vi "Initialize Waterfall Display for Octave.vi"(2 "colors":T2={"frame"=16763904, "plot"=52224, "background"=0}, 3 "display  bounds":T1={"left"=20, "top"=20, "width"=600, "heigth"=400} {"heigth" min=300; "width" min=400}, 4 "window title":string="Octave waterfall") -> (0 "error out":errorcluster, 1 "waterfall ref":refnum<vi>)   [LabVIEW 2017]
doc: "Initializes the waterfall display to display octave spectra and generates a waterfall reference to use to send data to this display or to close the display. This VI also specifies the title, colors and display bounds of the waterfall display. This VI does not open the waterfall display. The waterfall display opens when it receives its first data from Send Data to Waterfall for Octave VI."
uses:
  <vilib>/addons/Sound and Vibration/compatibility/Waterfall/subVIs/sv_Waterfall for Octave Global.vi
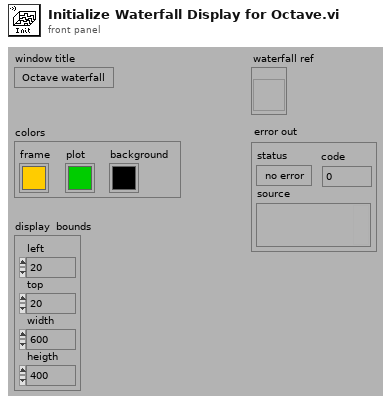
[diagram p1: front panel]
types:
  T1 = cluster{"left":i16, "top":i16, "width":i16, "heigth":i16}
  T2 = cluster{"frame":u32, "plot":u32, "background":u32}
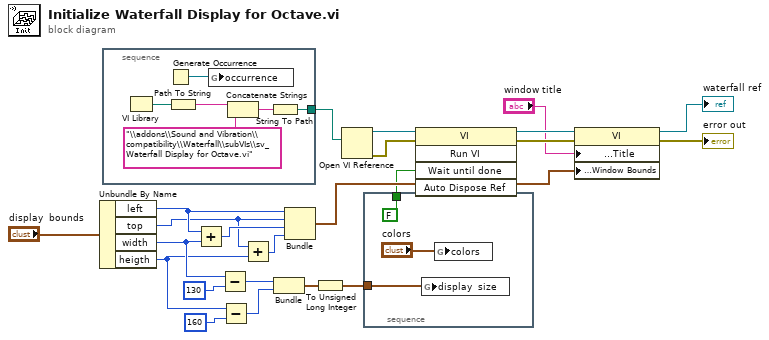
[diagram p0: block diagram]
diagram:
  n1 = Unbundle By Name("display  bounds") -> ("left"=w15:i16, "top"=w13:i16, "width"=w9:i16, "heigth"=w5:i16)
  n2 = stacked-sequence {
    tunnel: [w24] -> w1
    frame #0 {
      n3 = VI Library() -> (path=w25:path)
      n4 = Generate Occurrence() -> (w29:refnum<k4>)
      n5 = Path To String(path=w25) -> (string=w28:string)
      n6 = global write "sv_Waterfall for Octave Global.vi" "occurrence"(w29) -> ()
      n7 = Concatenate Strings(w28, "\\addons\\Sound and Vibration\\compatibility\\Waterfall\\subVIs\\sv_Waterfall Display for Octave.vi" ("Substring")) -> (w26:string)
      n8 = String To Path(string=w26) -> (path=w24:path)
    }
  }
  n9 = Add(x=w15, y=w9) -> (x+y=w14:i16)
  n10 = Subtract(x=w9, y=i16 130) -> (x-y=w7:i16)
  n11 = Subtract(x=w5, y=i16 160) -> (x-y=w4:i16)
  n12 = Add(x=w13, y=w5) -> (x+y=w12:i16)
  n13 = Bundle(w7, w4) -> (w11:cluster{i16, i16})  [unwired: 1 in]
  n14 = Bundle("left"=w15, "top"=w13, w14, w12) -> (w17:cluster{"left":i16, "top":i16, i16, i16})  [unwired: 1 in]
  n15 = To Unsigned Long Integer(number=w11) -> (unsigned 32bit integer=w10:cluster{u32, u32})
  n16 = Open VI Reference(vi path=w1) -> (vi reference=w23:refnum<vi>, error out=w22:errorcluster)  [unwired: 5 in]
  n17 = stacked-sequence {
    tunnel: w10 -> [w31]
    tunnel: [FALSE ("Wait until done")] -> w2
    frame #0 {
      n18 = global write "sv_Waterfall for Octave Global.vi" "display  size"(w31) -> ()
      n19 = global write "sv_Waterfall for Octave Global.vi" "colors"("colors") -> ()
    }
  }
  n20 = invoke class="VI" method="Run VI"(reference=w23, error in=w22, "Wait until done"=w2) -> (reference out=w20:refnum<vi>, error out=w21:errorcluster)  [unwired: 2 in, 3 out]
  n21 = property class="VI"(reference=w20, error in=w21, "Front Panel Window:Title"="window title", "Front Panel Window:Window Bounds"=w17) -> (reference out=→"waterfall ref":refnum<vi>, error out=→"error out":errorcluster)
